vi "ProbeStation.vi"() -> ()   [LabVIEW 2019]
panel:
  in  "SP Min Usable Z":dbl=4500.0
  in  "SP Comm Params":T1={"SP Error Debug"=FALSE, "LF as Return EOL"=TRUE}
  in  "SP LOCAL Comm Parameters":T2={"address"="localhost", "port"=5050, "SP TCP Cnx ID"=refnum, "mode (standard)"=enum."Immediate", "bytes to read"=300, "timeout (ms)"=1000000}
  in  "SP Local":bool
  out "SP Center of Rotation Y":dbl=105030.0
  out "SP Center of Rotation X":dbl=108495.0
  in  "SP REMOTE Comm Parameters":T3={"write delay(ms)"=500, "buffer is full loop multiplicity"=10, "read threshold check rate (ms)"=50}
  in  "SP Operation Parameters":T4={"SP Load Less Than Thr?"=TRUE, "SP Load Threshold (um)"=4800.0, "SP Current Location"={"X (um)"=20.0, "Y (um)"=20.0, "Z (um)"=20.0, "T (degree)"=20.0}, "SP Chuck Speeds"={"XY Speed (10-100%)"=10.0, "Z Speed (10-100%)"=10.0, "T Speed (10-100%)"=10.0}, "Manual Step Parameters"={"Step in X"=FALSE, "X S-Speed [µm/step]"=5.0, "Step in Y"=FALSE, "Y S-Speed [µm/step]"=5.0, "Step in Z"=FALSE, "Z S-Speed [µm/step]"=5.0, "Step in T"=FALSE, "T S-Speed [mdegree/step]"=5.0, "X Increase"=TRUE, "Y Increase?"=TRUE, "Z Increase?"=TRUE, "T Increase?"=TRUE}, "Z Stepper"={"UP/DOWN"=FALSE, "UP/DOWN Speed [µm/step]"=20, "SP Z Step"=FALSE}, "Z Heights Set"=FALSE, "SP Contact Search"={"Contact Circuit"=enum."1", "Speed [1000-10000]"=1000.0, "Start Height [µm]"=0.0, "Search Band [µm]"=100.0, "Use Contact Search?"=FALSE}} {"SP Contact Search"."Speed [1000-10000]" min=1000 max=10000; "SP Load Threshold (um)" format="%#_6f"}
  in  "SemiProbe VISA":refnum<visa-resource-name>
  in  "Probestation Configuration":T5(ring)
  in  "Z Heights and Arduino Edgesense":T6={"initial Z [µm]"=0.0, "search band [µm]"=0.0, "speed [µm/step]"=0.0, "overdrive [µm]"=0.0, "Use Overdrive?"=FALSE, "Seperation Distance [µm]"=30.0, "Contact Height [µm]"=30.0}
  out "Ref No.":i32
  out "Device ID Probe Station":i32=2
  # "Cambridge Alessi SemiAutomatic \nDDE Variables"
  # "SemiProbe SemiAutomatic\nOperation and Communication Variables"
  # "Of value set in the SP Navigation panel."
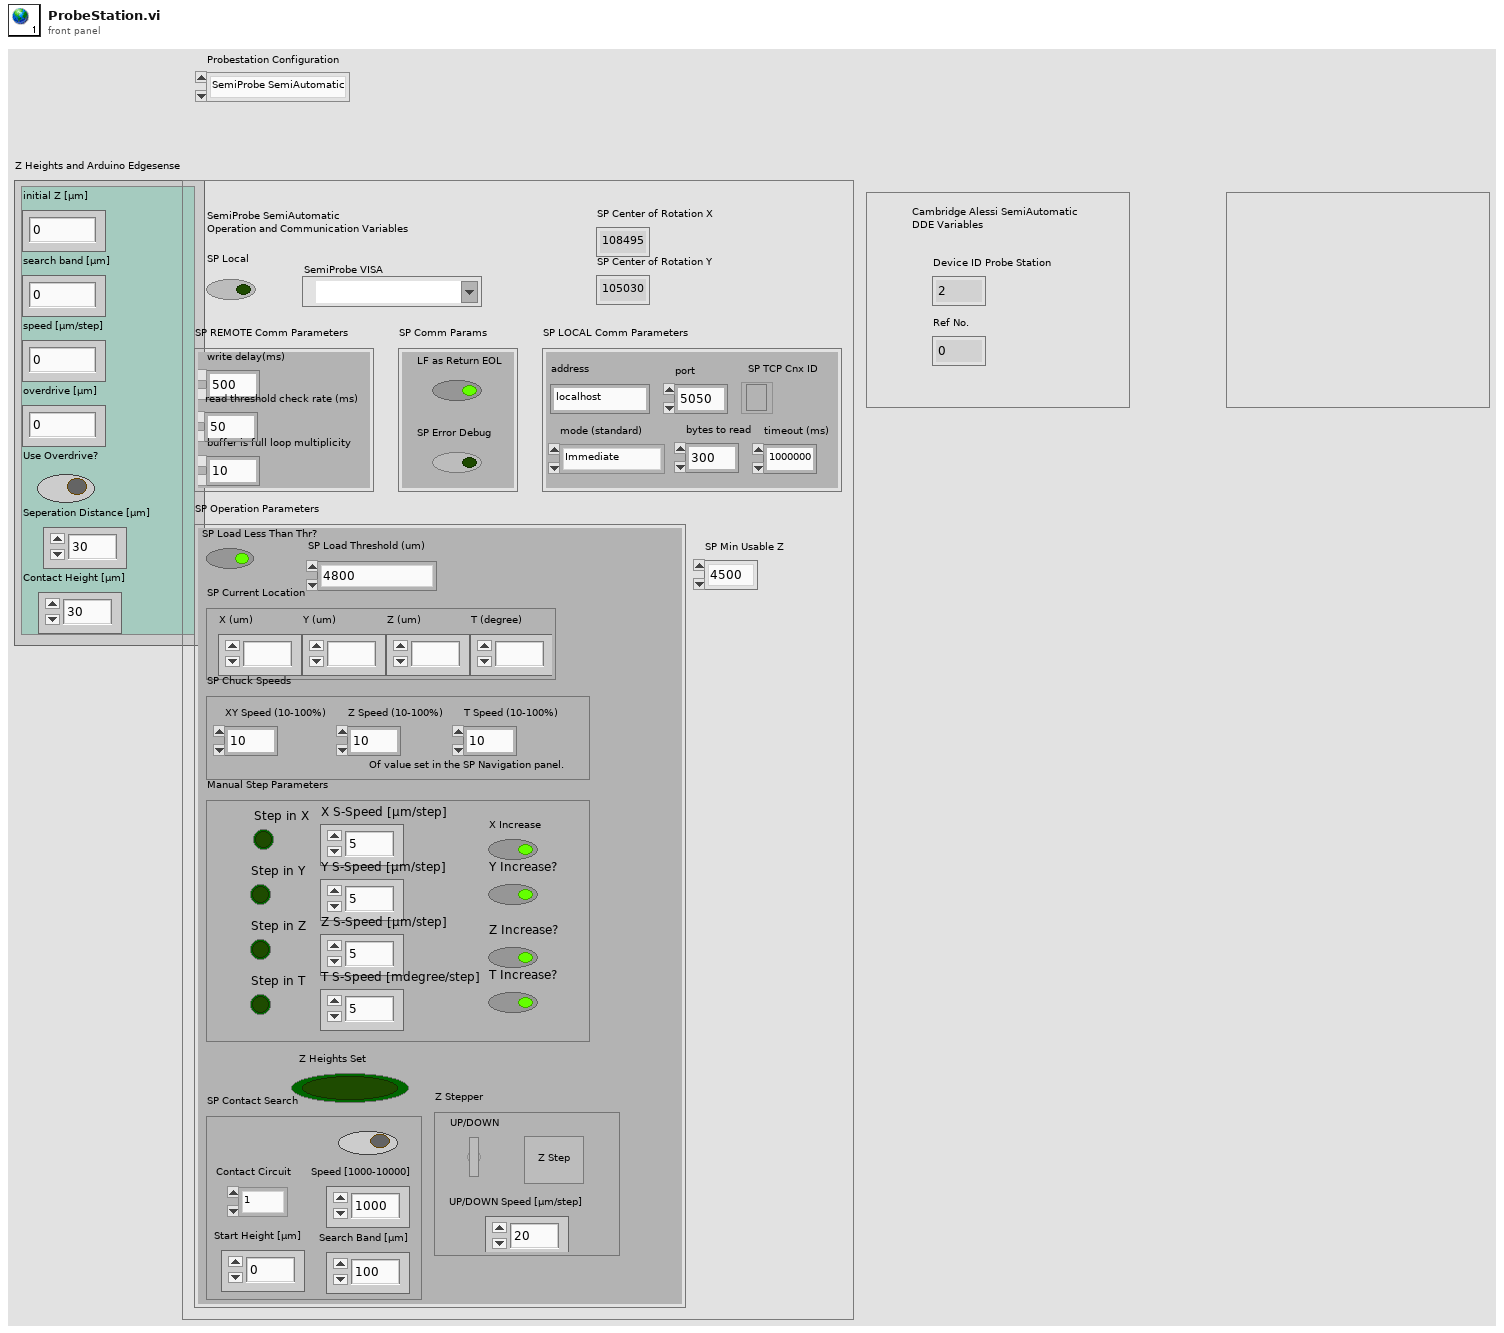
[diagram p1: front panel]
types:
  T1 = cluster{"SP Error Debug":bool, "LF as Return EOL":bool}
  T2 = cluster{"address":string, "port":i32, "SP TCP Cnx ID":refnum<k5>, "mode (standard)":enum16{"Standard", "Buffered", "CRLF", "Immediate"}, "bytes to read":i32, "timeout (ms)":i32}
  T3 = cluster{"write delay(ms)":i32, "buffer is full loop multiplicity":i32, "read threshold check rate (ms)":u32}
  T4 = cluster{"SP Load Less Than Thr?":bool, "SP Load Threshold (um)":dbl, "SP Current Location":cluster{"X (um)":ext, "Y (um)":ext, "Z (um)":ext, "T (degree)":ext}, "SP Chuck Speeds":cluster{"XY Speed (10-100%)":dbl, "Z Speed (10-100%)":dbl, "T Speed (10-100%)":dbl}, "Manual Step Parameters":cluster{"Step in X":bool, "X S-Speed [µm/step]":sgl, "Step in Y":bool, "Y S-Speed [µm/step]":sgl, "Step in Z":bool, "Z S-Speed [µm/step]":sgl, "Step in T":bool, "T S-Speed [mdegree/step]":sgl, "X Increase":bool, "Y Increase?":bool, "Z Increase?":bool, "T Increase?":bool}, "Z Stepper":cluster{"UP/DOWN":bool, "UP/DOWN Speed [µm/step]":i32, "SP Z Step":bool}, "Z Heights Set":bool, "SP Contact Search":cluster{"Contact Circuit":enum16{"12", "1", "2"}, "Speed [1000-10000]":sgl, "Start Height [µm]":sgl, "Search Band [µm]":sgl, "Use Contact Search?":bool}}
  T5 = enum16{"SemiProbe SemiAutomatic", "Cambridge Alessi SemiAutomatic", "Manual Probestation"}
  T6 = cluster{"initial Z [µm]":sgl, "search band [µm]":sgl, "speed [µm/step]":sgl, "overdrive [µm]":sgl, "Use Overdrive?":bool, "Seperation Distance [µm]":sgl, "Contact Height [µm]":sgl}
diagram:
